vi "shutdownComplete.vi"(8 "error in":errorcluster, 9 "Boiler Simulation Controls":refnum<vi>, 10 "Boiler Controls":refnum<vi>, 11 "Boiler Status Indicators":refnum<vi>) -> (0 "error out":errorcluster, 3 "elapsedTime":dbl)   [LabVIEW 2024]
uses:
  Controls/Boiler Simulation Controls.ctl
  Controls/Boiler Status Indicators.ctl
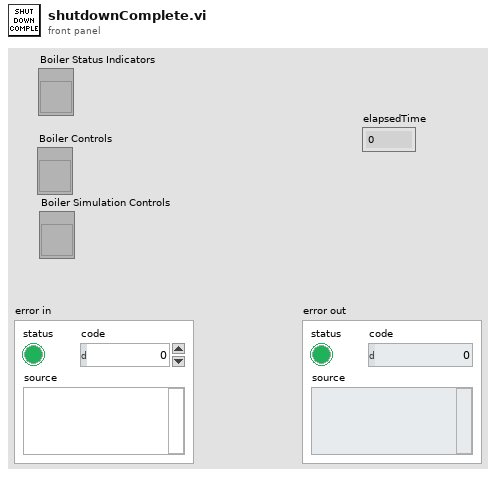
[diagram p1: front panel]
types:
  T1 = typedef "Boiler Status Indicators.ctl" = cluster{"Status":string, "Primary Fan":bool, "Natural Gas Valve":bool, "Pilot":bool, "Fuel Valve":bool, "Forced Draft Fan":bool, "Time Count":dbl}
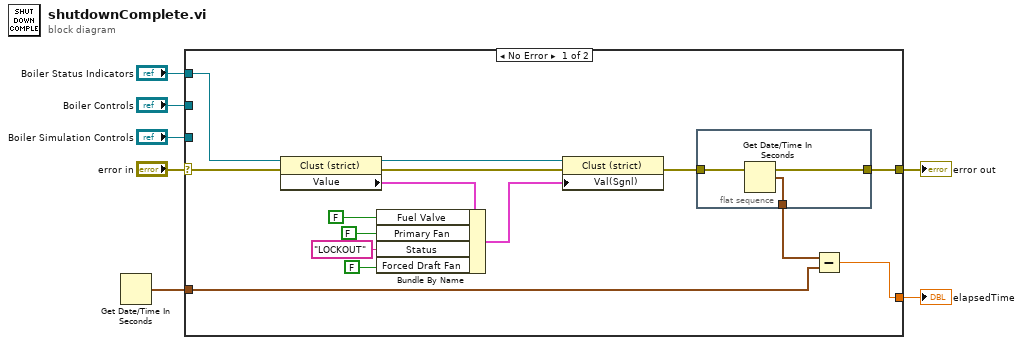
[diagram p0: block diagram]
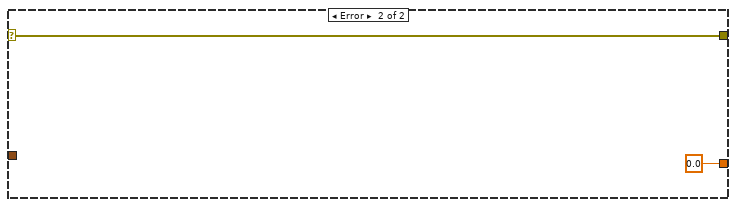
[diagram p2: hidden frame]
diagram:
  n1 = Get Date/Time In Seconds() -> (seconds since 1Jan1904=w1:timestamp)
  n2 = case shown="No Error" "error in" {
    selector: "error in" -> [w22 w26]
    tunnel: [w10 w26] -> w6
    tunnel: "Boiler Status Indicators" -> [w16 _]
    tunnel: "Boiler Controls" -> [_ _]
    tunnel: "Boiler Simulation Controls" -> [_ _]
    tunnel: [w13 0.0] -> w2
    tunnel: w1 -> [w12 _]
    frame No Error {
      n3 = property class="Clust (strict)"(reference=w16, error in=w22) -> (reference out=w19:refnum<vi>, error out=w18:errorcluster, "Value"=w21:T1)
      n4 = Bundle By Name(cluster=w21, "Fuel Valve"=FALSE ("Forced Draft Fan"), "Primary Fan"=FALSE, "Status"="LOCKOUT", "Forced Draft Fan"=FALSE) -> (w20:T1)
      n5 = property class="Clust (strict)"(reference=w19, error in=w18, "Val(Sgnl)"=w20) -> (error out=w11:errorcluster)  [unwired: 1 out]
      n6 = flat-sequence {
        tunnel: w11 -> [w24]
        tunnel: [w24] -> w10
        tunnel: [w23] -> w9
        frame #0 {
          n7 = Get Date/Time In Seconds() -> (seconds since 1Jan1904=w23:timestamp)
        }
      }
      n8 = Subtract(x=w9, y=w12) -> (x-y=w13:dbl)
    }
    frame Error {
    }
  }
  "error out" <- w6
  "elapsedTime" <- w2
